vi "ATF-Pump-Datalog Display NS creater.vi"(9 "Data FIFO Ref":T1, 11 "Queue in":refnum<queue>) -> ()   [LabVIEW 2022 SP3]
uses:
  RT Controls/ATF-Pump-Data FIFO.ctl
  RT Controls/ATF-Pump-DiplayPC comm ctrl.ctl
  <vilib>/dex/Stream Element Allocation Mode.ctl
  ATF-Pump-RT_Global_R.vi
  <resource>/objmgr/ni.dex.rc
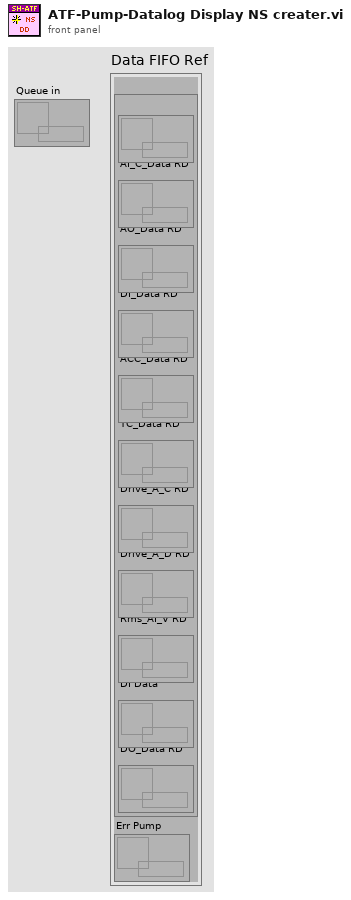
[diagram p1: front panel]
types:
  T1 = typedef "ATF-Pump-Data FIFO.ctl" = cluster{"RD":cluster{"AI_V_Data RD":refnum<queue>, "AI_C_Data RD":refnum<queue>, "AO_Data RD":refnum<queue>, "DI_Data RD":refnum<queue>, "ACC_Data RD":refnum<queue>, "TC_Data RD":refnum<queue>, "Drive_A_C RD":refnum<queue>, "Drive_A_D RD":refnum<queue>, "Rms_AI_V RD":refnum<queue>, "DI Data":refnum<queue>, "DO_Data RD":refnum<queue>}, "Err Pump":refnum<queue>}
  T2 = typedef "ATF-Pump-DiplayPC comm ctrl.ctl" = enum16{"Initialize", "Listen for UI Writer", "Send RT Data"}
  T3 = typedef "Stream Element Allocation Mode.ctl" = u32
  T4 = cluster{"Start DAQ":bool, "Stop DAQ":bool, "RT Stop":bool, "RT Exit":bool, "Start Seq":bool}
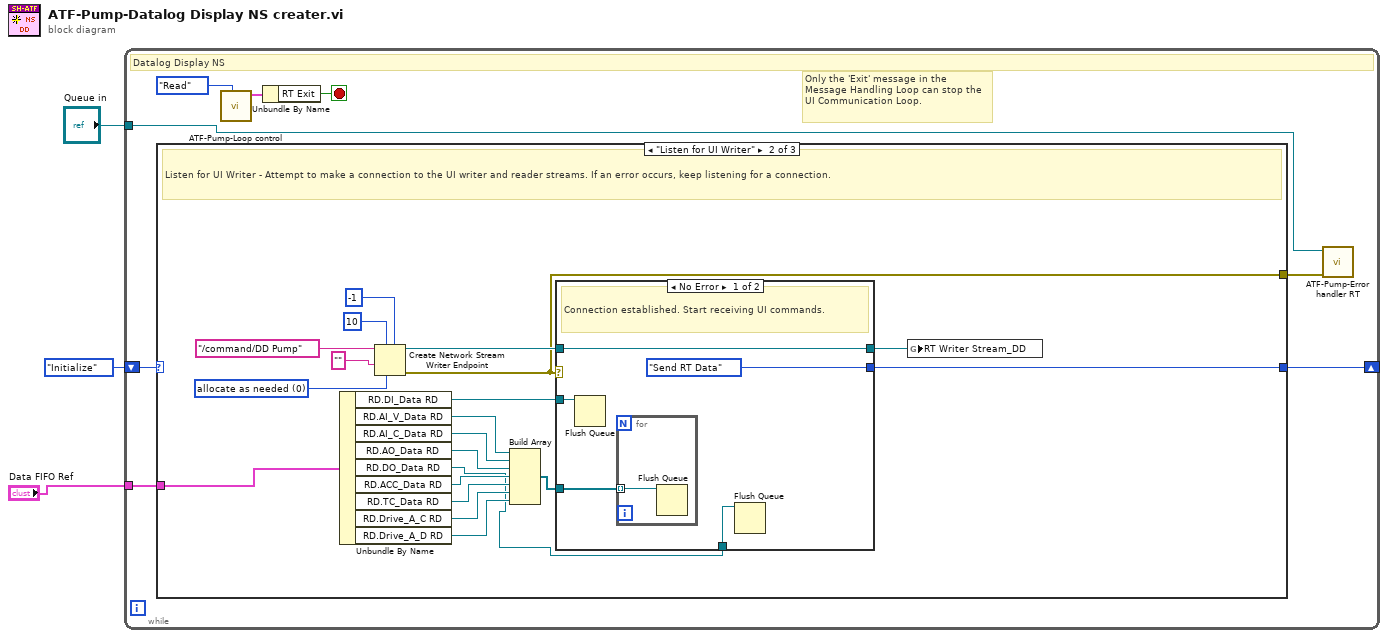
[diagram p0: block diagram]
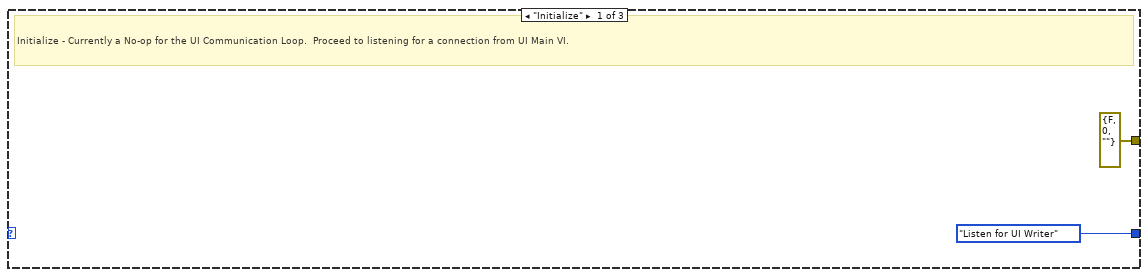
[diagram p2: hidden frame]
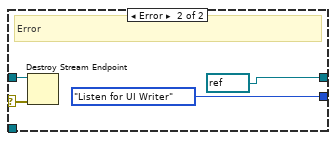
[diagram p3: hidden frame]
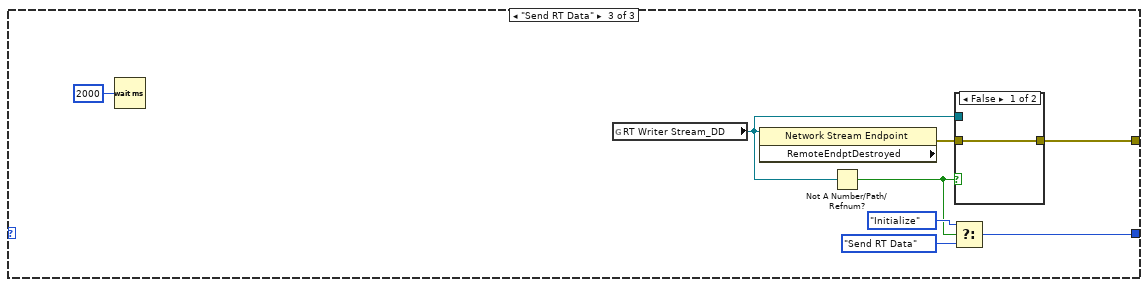
[diagram p4: hidden frame]
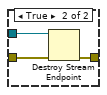
[diagram p5: hidden frame]
diagram:
  n1 = while {
    shift-right: [w11] -> _
    shift-left: ATF-Pump-DiplayPC_comm_ctrl."Initialize" -> [w10]
    tunnel: "Data FIFO Ref" -> [w9]
    tunnel: "Queue in" -> [w5]
    stop <- w6 stop-if-true
    # "Only the 'Exit' message in the  Message Handling Loop can stop the UI Communication Loop."
    # "Datalog Display NS"
    n2 = case shown="\"Listen for UI Writer\"" w10 {
      tunnel: [errorcluster {"status"=FALSE, "code"=0, "source"=""} ("error IO") w32 w44] -> w4
      tunnel: [ATF-Pump-DiplayPC_comm_ctrl."Listen for UI Writer" w31 w50] -> w11
      tunnel: w9 -> [_ w28 _]
      frame "Initialize" {
        # "Initialize - Currently a No-op for the UI Communication Loop.  Proceed to listening for a connection from UI Main VI."
      }
      frame "Listen for UI Writer" {
        w15 = T3 0 items=["allocate as needed", "pre-allocate"] ("element allocation mode")
        # "Listen for UI Writer - Attempt to make a connection to the UI writer and reader streams. If an error occurs, keep listening for a connection."
        n3 = Unbundle By Name(w28) -> ("RD.DI_Data RD"=w17:refnum<queue>, "RD.AI_V_Data RD"=w25:refnum<queue>, "RD.AI_C_Data RD"=w24:refnum<queue>, "RD.AO_Data RD"=w23:refnum<queue>, "RD.DO_Data RD"=w14:refnum<queue>, "RD.ACC_Data RD"=w22:refnum<queue>, "RD.TC_Data RD"=w21:refnum<queue>, "RD.Drive_A_C RD"=w20:refnum<queue>, "RD.Drive_A_D RD"=w19:refnum<queue>)
        n4 = Create Network Stream Writer Endpoint(5:-1 ("timeout in ms (-1)"), 6:w15, 7:10 ("writer buffer size"), 9:"" ("reader url"), 11:"/command/DD Pump" ("reader url")) -> (0:w32:errorcluster, 3:w33:refnum<k21>)  [unwired: 2 in]
        n5 = Build Array(w25, w24, w23, w22, w21, w20, w19) -> (w18:refnum<queue>[])
        n6 = case shown="No Error" w32 {
          selector: w32 -> [_ w41]
          tunnel: w33 -> [w37 w43]
          tunnel: [ATF-Pump-DiplayPC_comm_ctrl."Send RT Data" ATF-Pump-DiplayPC_comm_ctrl."Listen for UI Writer"] -> w31
          tunnel: [w37 refnum<k21> refnum ("reader url")] -> w26
          tunnel: w18 -> [w36 _]
          tunnel: w17 -> [w35 _]
          tunnel: w14 -> [w34 _]
          frame No Error {
            # "Connection established. Start receiving UI commands."
            n7 = Flush Queue(queue=w35) -> ()  [unwired: 1 in, 3 out]
            n8 = for {
              tunnel: w36 -> [w39] mode=indexing
              n9 = Flush Queue(queue=w39) -> ()  [unwired: 1 in, 3 out]
            }
            n10 = Flush Queue(queue=w34) -> ()  [unwired: 1 in, 3 out]
          }
          frame Error {
            # "Error"
            n11 = Destroy Stream Endpoint(8:w41, 11:w43) -> ()  [unwired: 1 out]
          }
        }
        n12 = global write "ATF-Pump-RT_Global_R.vi" "RT Writer Stream_DD"(w26) -> ()
      }
      frame "Send RT Data" {
        n13 = Wait (ms)(milliseconds to wait=u32 2000) -> ()  [unwired: 1 out]
        n14 = global read "ATF-Pump-RT_Global_R.vi" "RT Writer Stream_DD"() -> (w46:refnum<k21>)
        n15 = property class="Network Stream Endpoint" props=["RemoteEndptDestroyed"](reference=w46) -> (error out=w45:errorcluster)  [unwired: 1 in, 2 out]
        n16 = Not A Number/Path/Refnum?(number/path/refnum=w46) -> (NaN/Path/Refnum?=w47:bool)
        n17 = Select(t=ATF-Pump-DiplayPC_comm_ctrl."Initialize", s=w47, f=ATF-Pump-DiplayPC_comm_ctrl."Send RT Data") -> (s? t:f=w50:T2)
        n18 = case shown="False" w47 {
          tunnel: w46 -> [_ w55]
          tunnel: w45 -> [w52 w54]
          tunnel: [w52 w53] -> w44
          frame False {
          }
          frame True {
            n19 = Destroy Stream Endpoint(8:w54, 11:w55) -> (0:w53:errorcluster)
          }
        }
      }
    }
    n20 = call "ATF-Pump-Loop control.vi"("Action"=enum16{"Init", "Write", "Read"}."Read") -> ("Loop Control out"=w8:T4)  [unwired: 9 in, 1 out]
    n21 = Unbundle By Name(w8) -> ("RT Exit"=w6:bool)
    n22 = call "ATF-Pump-Error handler RT.vi"("error in"=w4, "Message Queue"=w5) -> ()  [unwired: 8 in, 2 out]
  }
